vi "Revision Query.vi"(8 "error in (no error)":errorcluster, 11 "VISA resource name":refnum<visa-resource-name>) -> (0 "error out":errorcluster, 1 "Instrument Firmware Revision":string, 2 "Instrument Driver Revision":string, 3 "VISA resource name out":refnum<visa-resource-name>)   [LabVIEW 2020, in "RIGOL DP1000 Series.lvlib"]
doc: "Queries the current instrument firmware revision and instrument driver revision.\n\nRefer to the Readme file for detailed driver information including modification history."
uses:
  <instrlib>/RIGOL DP1000 Series/RIGOL DP1000 Series.lvlib
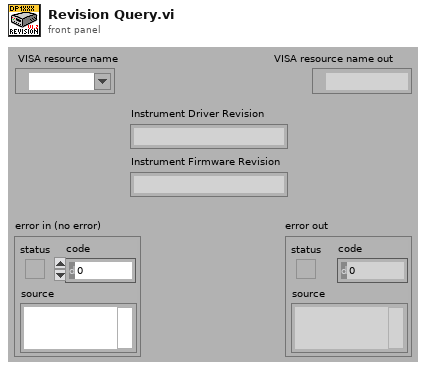
[diagram p1: front panel]
types:
  T1 = enum32{"invalid app kind", "Development System", "Run Time System", "Student Edition", "Embedded LabVIEW", "Evaluation", "Custom"}
  T2 = cluster{"Major":u16, "Minor":u16, "Fix":u16, "Build":u16}
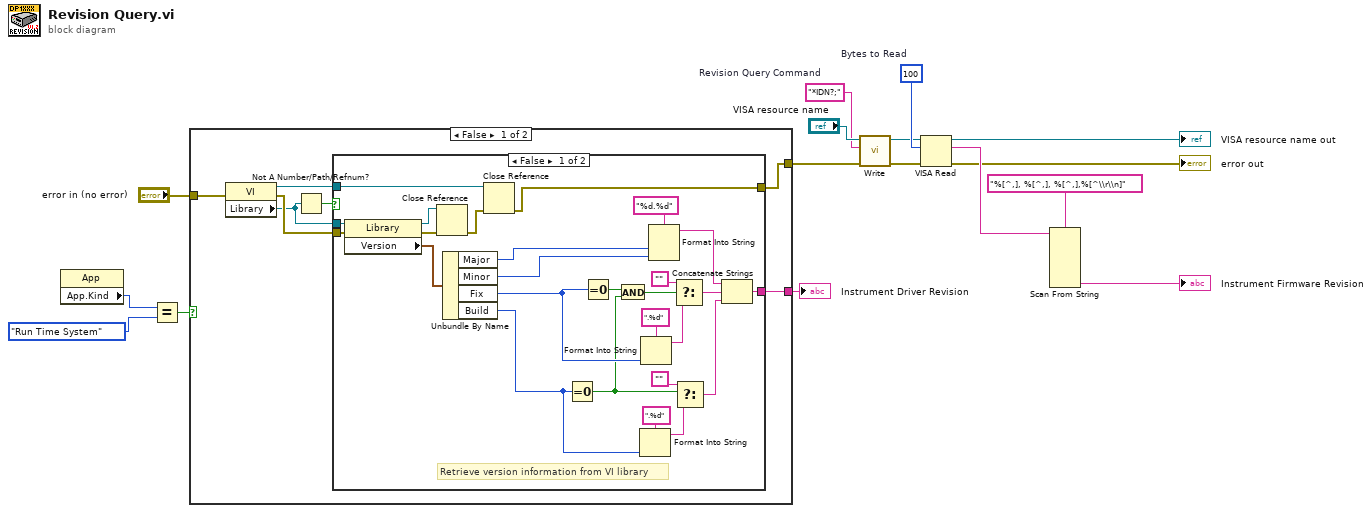
[diagram p0: block diagram]
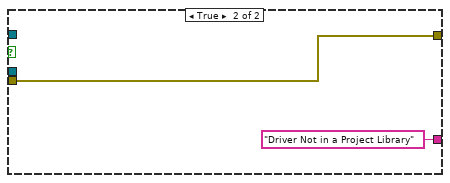
[diagram p2: hidden frame]
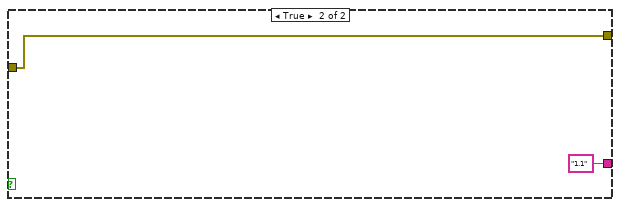
[diagram p3: hidden frame]
diagram:
  w1 = "*IDN?;"  # Revision Query Command
  w15 = u32 100  # Bytes to Read
  n1 = property class="App"() -> ("App.Kind"=w9:T1)  [unwired: 2 in, 2 out]
  n2 = Equal?(x=w9, y=T1."Run Time System" ("Application:Kind")) -> (x = y?=w10:bool)
  n3 = case shown="False" w10 {
    tunnel: [w19 "1.1"] -> w12
    tunnel: "error in (no error)" -> [w18 w52]
    tunnel: [w17 w52] -> w2
    frame False {
      n4 = property class="VI"(error in=w18) -> (reference out=w23:refnum<vi>, error out=w22:errorcluster, "Library"=w21:refnum<vi>)  [unwired: 1 in]
      n5 = Not A Number/Path/Refnum?(number/path/refnum=w21) -> (NaN/Path/Refnum?=w20:bool)
      n6 = case shown="False" w20 {
        tunnel: w23 -> [w46 _]
        tunnel: w22 -> [w31 w51]
        tunnel: [w26 w51] -> w17
        tunnel: [w25 "Driver Not in a Project Library"] -> w19
        tunnel: w21 -> [w24 _]
        frame False {
          # "Retrieve version information from VI library"
          n7 = property class="Library"(reference=w24, error in=w31) -> (reference out=w48:refnum<vi>, error out=w49:errorcluster, "Version"=w45:T2)
          n8 = Close Reference(reference=w48, error in (no error)=w49) -> (error out=w47:errorcluster)
          n9 = Unbundle By Name(w45) -> ("Major"=w34:u16, "Minor"=w33:u16, "Fix"=w30:u16, "Build"=w32:u16)
          n10 = Close Reference(reference=w46, error in (no error)=w47) -> (error out=w26:errorcluster)
          n11 = Equal To 0?(x=w32) -> (x = 0?=w28:bool)
          n12 = Equal To 0?(x=w30) -> (x = 0?=w29:bool)
          n13 = And(x=w29, y=w28) -> (x .and. y?=w27:bool)
          n14 = Format Into String(format string=".%d", w32) -> (resulting string=w38:string)  [unwired: 2 in, 1 out]
          n15 = Format Into String(format string=".%d", w30) -> (resulting string=w42:string)  [unwired: 2 in, 1 out]
          n16 = Format Into String(format string="%d.%d", w34, w33) -> (resulting string=w40:string)  [unwired: 2 in, 1 out]
          n17 = Select(t="", s=w27, f=w42) -> (s? t:f=w39:string)
          n18 = Select(t="", s=w28, f=w38) -> (s? t:f=w35:string)
          n19 = Concatenate Strings(w40, w39, w35) -> (w25:string)
        }
        frame True {
        }
      }
    }
    frame True {
    }
  }
  "Instrument Driver Revision" <- w12
  n20 = call <instrlib>:"Write.vi"("error in (no error)"=w2, "Write Buffer (\"\")"=w1, "VISA resource name"="VISA resource name") -> ("error out"=w5:errorcluster, "VISA resource name out"=w4:refnum<visa-resource-name>)  [unwired: 7 in]
  n21 = VISA Read(VISA resource name=w4, byte count=w15, error in (no error)=w5) -> (VISA resource name out=→"VISA resource name out":refnum<visa-resource-name>, read buffer=w14:string, error out=→"error out":errorcluster)  [unwired: 1 out]
  n22 = Scan From String(format string="%[^,], %[^,], %[^,],%[^\\r\\n]", input string=w14) -> (output 4=→"Instrument Firmware Revision":string)  [unwired: 2 in, 10 out]
